vi "MTEC_Async_Init.vi"(0 "object in":refnum<class "MTEC_Async.lvclass">, 4 "SW Buffer Size":i32, 5 "error in (no error)":errorcluster, 8 "Sample Rate (Hz)":dbl=10.0) -> (14 "object out":refnum<class "MTEC_Async.lvclass">, 19 "error out":errorcluster)   [LabVIEW 2019, in "MTEC_Async.lvclass"]
uses:
  MTEC_Async.lvclass
  TEC LabVIEW Control Software v0.14/Source/LV Source/[meerstetter engineering TE Cooling]/TypeDefs/meTEC_ID 1200_Temperature is Stable.ctl
  TEC LabVIEW Control Software v0.14/Source/LV Source/[meerstetter engineering TE Cooling]/TypeDefs/meTEC_ID 104_Device Status.ctl
  MTEC_Async.lvclass/MTEC_Async.ctl
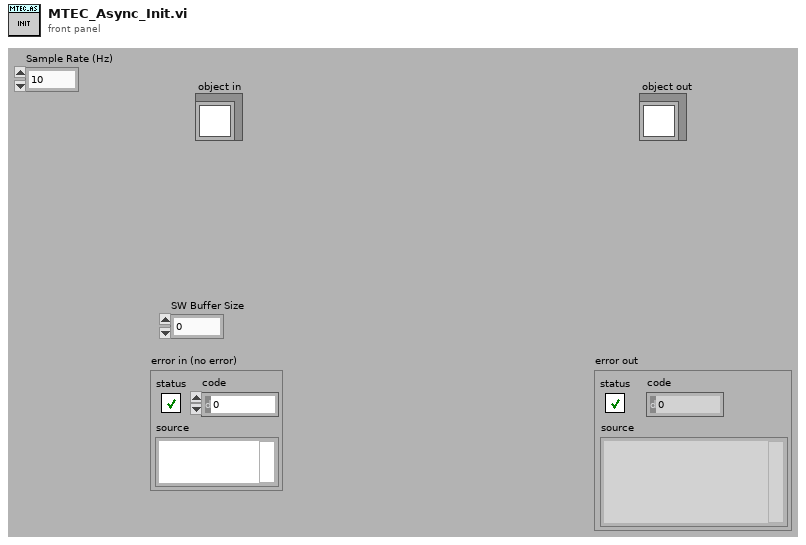
[diagram p1: front panel]
types:
  T1 = cluster{"Message":string, "Message Data":variant}
  T2 = enum32{"Invalid", "Standard", "Closed", "Hidden", "Minimized", "Maximized"}
  T3 = typedef "meTEC_ID 1200_Temperature is Stable.ctl" = i32
  T4 = typedef "meTEC_ID 104_Device Status.ctl" = i32
  T5 = cluster{"current time":timestamp, "DataOut":cluster{"meTEC_CH2_Temperature Stability":T3, "meTEC_CH2_Act. Output Current [A]":dbl, "meTEC_CH2_Act. Output Voltage [V]":dbl, "meTEC_CH2_Object Temperature [°C]":dbl, "meTEC_CH2_Sink Temperature [°C]":dbl, "meTEC_CH1_Error Parameter":i32, "meTEC_CH1_Error Instance":i32, "meTEC_CH1_Error No.":i32, "meTEC_CH1_Device Status":T4, "meTEC_CH1_Temperature Stability":T3, "meTEC_CH1_Act. Output Current [A]":dbl, "meTEC_CH1_Act. Output Voltage [V]":dbl, "meTEC_CH1_Object Temperature [°C]":dbl, "meTEC_CH1_Sink Temperature [°C]":dbl}}
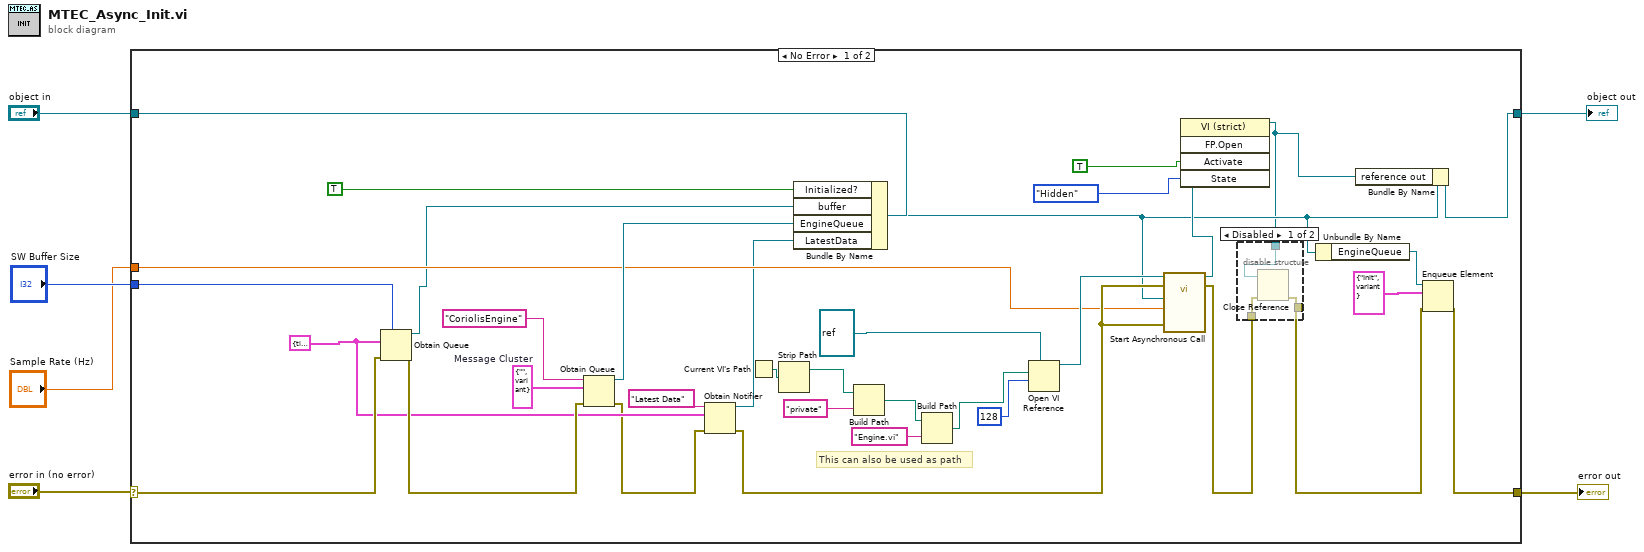
[diagram p0: block diagram]
diagram:
  n1 = case shown="No Error" "error in (no error)" {
    selector: "error in (no error)" -> [w40 w45]
    tunnel: "object in" -> [w41 w46]
    tunnel: [w8 w46] -> w5
    tunnel: [w9 w45] -> w3
    tunnel: "SW Buffer Size" -> [w38 _]
    tunnel: "Sample Rate (Hz)" -> [w19 _]
    frame No Error {
      w37 = T1 {"Message"="", "Message Data"=variant}  # Message Cluster
      w33 = T5 {"current time"=timestamp(0 s since 1904-01-01), "DataOut"={"meTEC_CH2_Temperature Stability"=0, "meTEC_CH2_Act. Output Current [A]"=0.0, "meTEC_CH2_Act. Output Voltage [V]"=0.0, "meTEC_CH2_Object Temperature [°C]"=0.0, "meTEC_CH2_Sink Temperature [°C]"=0.0, "meTEC_CH1_Error Parameter"=0, "meTEC_CH1_Error Instance"=0, "meTEC_CH1_Error No."=0, "meTEC_CH1_Device Status"=0, "meTEC_CH1_Temperature Stability"=0, "meTEC_CH1_Act. Output Current [A]"=0.0, "meTEC_CH1_Act. Output Voltage [V]"=0.0, "meTEC_CH1_Object Temperature [°C]"=0.0, "meTEC_CH1_Sink Temperature [°C]"=0.0}}
      # "This can also be used as path"
      n2 = Obtain Queue(max queue size (-1, unlimited)=w38, element data type=w33, error in (no error)=w40) -> (queue out=w15:refnum<queue>, error out=w36:errorcluster)  [unwired: 2 in, 1 out]
      n3 = Obtain Queue(name (unnamed)="CoriolisEngine", element data type=w37, error in (no error)=w36) -> (queue out=w34:refnum<queue>, error out=w31:errorcluster)  [unwired: 2 in, 1 out]
      n4 = Obtain Notifier(name (unnamed)="Latest Data", notification data type=w33, error in (no error)=w31) -> (notifier out=w14:refnum<notifier>, error out=w24:errorcluster)  [unwired: 1 in, 1 out]
      n5 = Current VI's Path() -> (path=w28:path)
      n6 = Strip Path(path=w28) -> (stripped path=w29:path)  [unwired: 1 out]
      n7 = Bundle By Name(cluster=w41, "Initialized?"=TRUE ("InstrumentInitialized?"), "buffer"=w15, "EngineQueue"=w34, "LatestData"=w14) -> (w13:refnum<class "MTEC_Async.lvclass">)
      n8 = Build Path(base path=w29, name or relative path="private") -> (appended path=w30:path)
      n9 = Build Path(base path=w30, name or relative path="Engine.vi") -> (appended path=w20:path)
      n10 = Open VI Reference(type specifier VI Refnum (for type only)=refnum<vi> refnum, vi path=w20, options=128) -> (vi reference=w23:refnum<vi>)  [unwired: 3 in, 1 out]
      n11 = call-by-ref "Start Asynchronous Call"(reference=w23, error in=w24, "object in"=w13, "Sample Rate (Hz)"=w19, 5:"error in (no error)"=w24) -> (reference out=w16:refnum<vi>, error out=w22:errorcluster)  [unwired: 15 in, 2 out]
      n12 = invoke class="VI (strict)" method="FP.Open"(reference=w16, "Activate"=TRUE ("Activate?"), "State"=T2."Hidden") -> (reference out=w7:refnum<vi>)  [unwired: 2 in, 4 out]
      n13 = disable-structure shown="Disabled" {
        disable-tunnel: w22 -> [w44 _]
        disable-tunnel: w7 -> [w43 _]
        disable-tunnel: [w42 _] -> w10
        frame Disabled {
          n14 = Close Reference(reference=w43, error in (no error)=w44) -> (error out=w42:errorcluster)
        }
        frame Enabled {
        }
      }
      n15 = Unbundle By Name(w13) -> ("EngineQueue"=w12:refnum<queue>)
      n16 = Bundle By Name(cluster=w13, "reference out"=w7) -> (w8:refnum<class "MTEC_Async.lvclass">)
      n17 = Enqueue Element(queue=w12, element=T1 {"Message"="Init", "Message Data"=variant}, error in (no error)=w10) -> (error out=w9:errorcluster)  [unwired: 1 in, 2 out]
    }
    frame Error {
    }
  }
  "object out" <- w5
  "error out" <- w3
